vi "Full Complex Matrix Cholesky Factorization.vi"(0 "A":T1) -> (1 "Cholesky R":T1, 2 "error":i32)   [LabVIEW 2017, in "NI_AALBase.lvlib"]
uses:
  NI_AALBase.lvlib
  ComplexMatrix.ctl
  <resource>/lvanlys.dll
  NI_Matrix.lvlib
panel:
  # "Full Complex Matrix Cholesky Factorization"
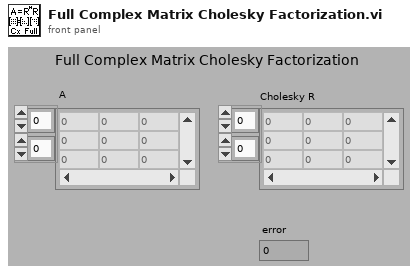
[diagram p1: front panel]
types:
  T1 = typedef "NI_Matrix.lvlib/ComplexMatrix.ctl" = cdb[][]
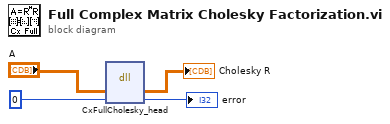
[diagram p0: block diagram]
diagram:
  n1 = dll-call lib="C:/Program Files (x86)/National Instruments/LabVIEW 2017/resource/lvanlys.*" fn="CxFullCholesky_head"("A"="A", "error"=0) -> ("A"=→"Cholesky R":T1, "error"=→"error":i32)  [unwired: 4 in, 2 out]
